vi "ASI_Standalone.vi"() -> ()   [LabVIEW 2011]
panel:
  in  "end":bool
  in  "z":dbl(slide) scale=0.0..10.0
  in  "y [mm]":dbl(slide) scale=-10.0..20.0
  in  "x [mm]":dbl(slide) scale=-10.0..20.0
  in  "VISA resource name":refnum<visa-resource-name>
  # "close port"
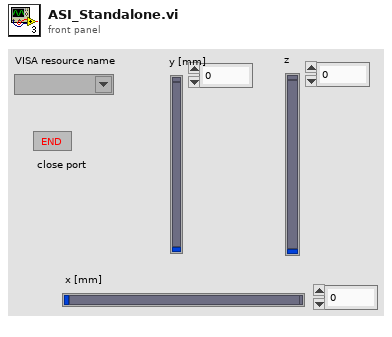
[diagram p1: front panel]
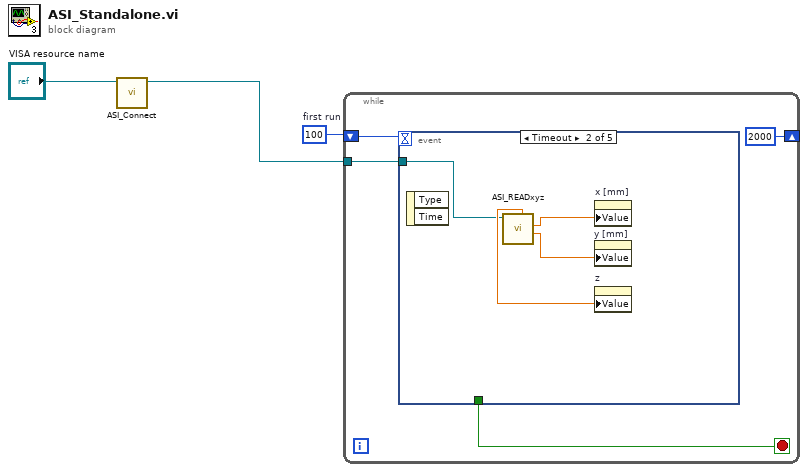
[diagram p0: block diagram]
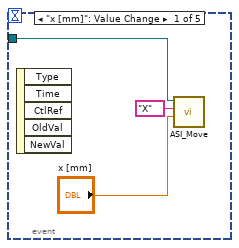
[diagram p2: hidden frame]
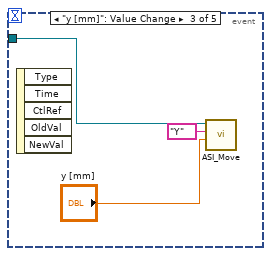
[diagram p3: hidden frame]
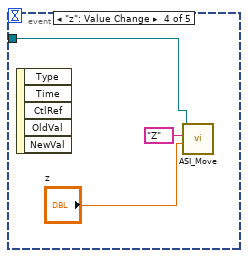
[diagram p4: hidden frame]
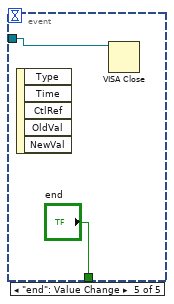
[diagram p5: hidden frame]
diagram:
  w1 = 100  # first run
  n1 = call "ASI_Connect.vi"("VISA resource name"="VISA resource name") -> ("VISA resource name out"=w2:refnum<visa-resource-name>)  [unwired: 9 in, 1 out]
  n2 = while {
    tunnel: w2 -> [w6]
    shift-right: [2000] -> _
    shift-left: w1 -> [w5]
    stop <- w7 stop-if-true
    n3 = event shown="[1] Timeout" {
      selector: _ -> [_ _ _ _ _]
      dyn-events: _ -> [_ _ _ _ _]
      timeout: w5 -> [_ _ _ _ _]
      tunnel: [_ _ _ _ "end"] -> w7
      tunnel: w6 -> [w10 w11 w17 w18 w21]
      event "x [mm]": Value Change {
        n4 = event-data() -> ()  [unwired: 1 in, 5 out]
        n5 = call "ASI_Move.vi"("Position [mm]"="x [mm]", "Axis"="X", "VISA resource name"=w10) -> ()  [unwired: 7 in, 2 out]
      }
      event Timeout {
        n6 = event-data() -> ()  [unwired: 1 in, 2 out]
        n7 = call "ASI_READxyz.vi"("VISA resource name"=w11) -> ("y [mm]"=w13:dbl, "x [mm]"=w12:dbl, "z [mm]"=w14:dbl)  [unwired: 6 in, 2 out]
        n8 = property on="x [mm]" class="Slide (strict)"("Value"=w12) -> ()  [unwired: 2 in, 2 out]
        n9 = property on="y [mm]" class="Slide (strict)"("Value"=w13) -> ()  [unwired: 2 in, 2 out]
        n10 = property on="z" class="Slide (strict)"("Value"=w14) -> ()  [unwired: 2 in, 2 out]
      }
      event "y [mm]": Value Change {
        n11 = event-data() -> ()  [unwired: 1 in, 5 out]
        n12 = call "ASI_Move.vi"("Position [mm]"="y [mm]", "Axis"="Y", "VISA resource name"=w17) -> ()  [unwired: 7 in, 2 out]
      }
      event "z": Value Change {
        n13 = event-data() -> ()  [unwired: 1 in, 5 out]
        n14 = call "ASI_Move.vi"("Position [mm]"="z", "Axis"="Z", "VISA resource name"=w18) -> ()  [unwired: 7 in, 2 out]
      }
      event "end": Value Change {
        n15 = event-data() -> ()  [unwired: 1 in, 5 out]
        n16 = VISA Close(VISA resource name=w21) -> ()  [unwired: 1 in, 1 out]
      }
    }
  }
